vi "Read Bytes.vi"   [LabVIEW 2019, in "LabPack.lvlib" / "Reader.lvclass"]
doc: "Reads, but does not decode, bytes from the MessagePack data. This is used to read strings, binary, and extension data. Use the Begin and End VIs for the various types with this VI to decode the bytes from the MessagePack format."
uses:
  Reader.lvclass
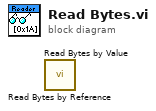
[diagram p0: block diagram]
diagram:
  n1 = call "Read Bytes by Reference.vi"() -> ()  [unwired: 9 in, 3 out]
  n2 = call "Read Bytes by Value.vi"() -> ()  [unwired: 9 in, 3 out]
